vi "RestURLFGV.vi"(7 "Action":T1, 8 "error in (no error)":errorcluster, 10 "URL":string) -> (0 "error out":errorcluster, 2 "URL":string)   [LabVIEW 2015, in "RestApi.lvlib"]
uses:
  RestApi.lvlib
  FGVAction.ctl
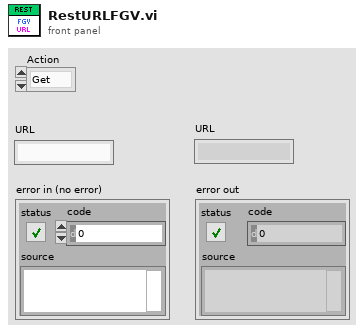
[diagram p1: front panel]
types:
  T1 = typedef "FGVAction.ctl" = enum16{"Get", "Set"}
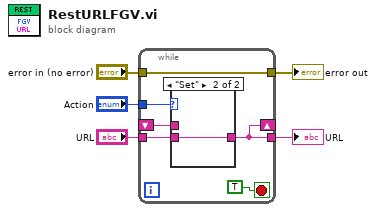
[diagram p0: block diagram]
diagram:
  n1 = while {
    shift-right: [w8] -> _
    shift-left: _ -> [w7]
    tunnel: "Action" -> [w10]
    tunnel: "URL" -> [w9]
    tunnel: [w8] -> w3
    tunnel: [w6] -> w1
    tunnel: "error in (no error)" -> [w6]
    stop <- TRUE stop-if-true
    n2 = case shown="\"Set\"" w10 {
      tunnel: [w12 w13] -> w8
      tunnel: w9 -> [_ w13]
      tunnel: w7 -> [w12 _]
      frame "Get", Default {
      }
      frame "Set" {
      }
    }
  }
  "URL" <- w3
  "error out" <- w1
